vi "image properties.vi"(0 "Image in":T2, 5 "error in (no error)":errorcluster) -> (11 "Image Type":T1 items=["Grayscale (U8)", "Grayscale (I16)", "Grayscale (SGL)", "Complex (CSG)", "RGB (U32)", "HSL (U32)", "RGB (U64)", "Grayscale (U16)"], 13 "Image Name":string, 14 "Image out":T2, 15 "Pixel Pointer out":u64, 16 "Line Width":i32, 17 "X Resolution":i32, 18 "Y Resolution":i32, 19 "error out":errorcluster)   [LabVIEW 2024, in "Vision.lvlib"]
uses:
  Vision.lvlib
  <vilib>/vision/Image Controls.llb/IMAQ Image.ctl
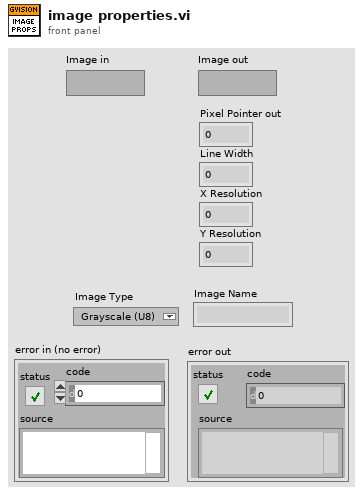
[diagram p1: front panel]
types:
  T1 = typedef "Image Type" = u32
  T2 = typedef "IMAQ Image.ctl" = refnum<image>
  T3 = enum32{"Map Pixel Pointer", "Unmap Pixel Pointer", "Get Pixels Infos"}
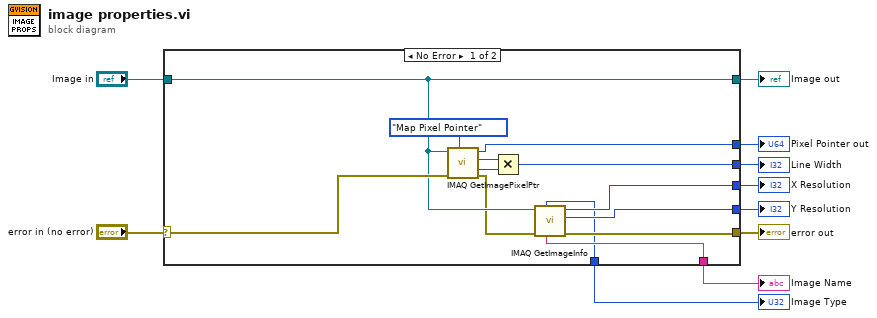
[diagram p0: block diagram]
diagram:
  n1 = case shown="No Error" "error in (no error)" {
    selector: "error in (no error)" -> [w20 w25]
    tunnel: "Image in" -> [w17 w24]
    tunnel: [w13 w25] -> w8
    tunnel: [w17 w24] -> w7
    tunnel: [w19 _] -> w6
    tunnel: [w18 _] -> w5
    tunnel: [w15 _] -> w4
    tunnel: [w14 _] -> w3
    tunnel: [w12 _] -> w2
    tunnel: [w11 _] -> w1
    frame No Error {
      n2 = call "IMAQ GetImagePixelPtr"("Function"=T3."Map Pixel Pointer", "error in (no error)"=w20, "Image"=w17) -> ("error out"=w16:errorcluster, "Pixel Size (Bytes)"=w21:i32, "LineWidth(Pixels)"=w22:i32, "Pixel Pointer out"=w19:u64)  [unwired: 3 in, 2 out]
      n3 = Multiply(x=w22, y=w21) -> (x*y=w18:i32)
      n4 = call "IMAQ GetImageInfo"("error in (no error)"=w16, "Image"=w17) -> ("error out"=w13:errorcluster, "Y Resolution"=w14:i32, "X Resolution"=w15:i32, "Image Name"=w12:string, "Image Type"=w11:T1)  [unwired: 2 in, 3 out]
    }
    frame Error {
    }
  }
  "Image out" <- w7
  "error out" <- w8
  "Pixel Pointer out" <- w6
  "Line Width" <- w5
  "X Resolution" <- w4
  "Y Resolution" <- w3
  "Image Name" <- w2
  "Image Type" <- w1
